vi "Read Full Name.vi"(8 "error in (no error)":errorcluster, 11 "Instrument Information in":refnum<class "Instrument.lvclass">) -> (0 "error out":errorcluster, 2 "Full Name":string, 3 "Instrument Information out":refnum<class "Instrument.lvclass">)   [LabVIEW 2015, in "Item Actor.lvlib" / "Instrument.lvclass"]
uses:
  Instrument.lvclass
  Instrument.lvclass/Instrument.ctl
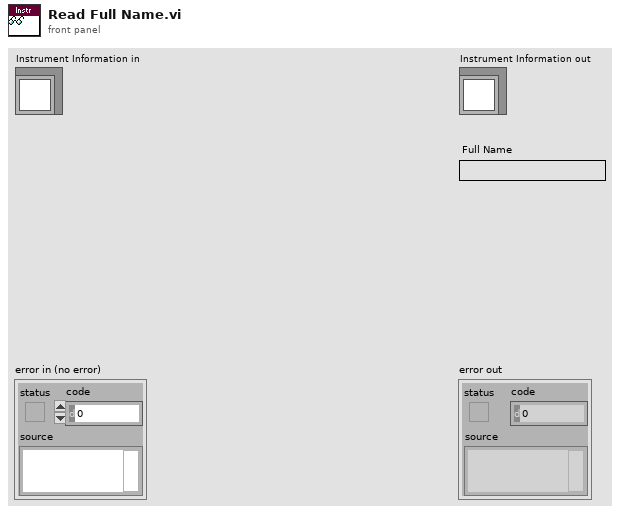
[diagram p1: front panel]
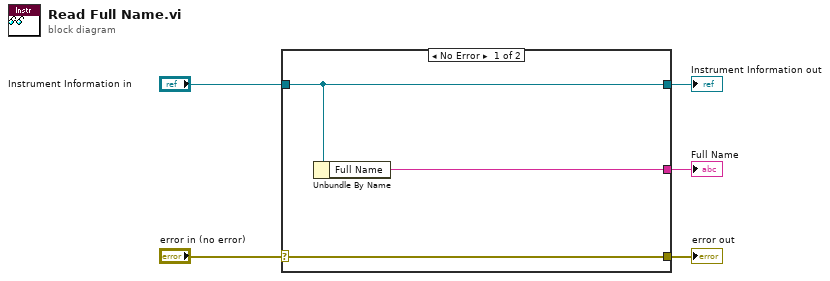
[diagram p0: block diagram]
diagram:
  n1 = case shown="No Error" "error in (no error)" {
    selector: "error in (no error)" -> [w8 w9]
    tunnel: [w8 w9] -> w4
    tunnel: [w7 w10] -> w2
    tunnel: "Instrument Information in" -> [w7 w10]
    tunnel: [w6 _] -> w1
    frame No Error {
      n2 = Unbundle By Name(w7) -> ("Full Name"=w6:string)
    }
    frame Error {
    }
  }
  "error out" <- w4
  "Instrument Information out" <- w2
  "Full Name" <- w1
